vi "detElementContents.vi"(8 "error in (no error)":errorcluster, 10 "XMLString in":string, 11 "Element in":refnum<class "XMLParser.lvclass">) -> (0 "error out":errorcluster, 3 "Element out":refnum<class "XMLParser.lvclass">)   [LabVIEW 2014, in "XML.lvlib" / "XMLParser.lvclass"]
doc: "This method retrieves XML element contents of the XML input string."
uses:
  <userlib>/Common/XML/XMLParser/XMLParser.lvclass
  <userlib>/Common/XML/XMLParser/XMLParser.lvclass/XMLParser.ctl
  <vilib>/Utility/error.llb/Trim Whitespace.vi
  <userlib>/Common/XML/XMLAttributeParser/XMLAttributeParser.lvclass
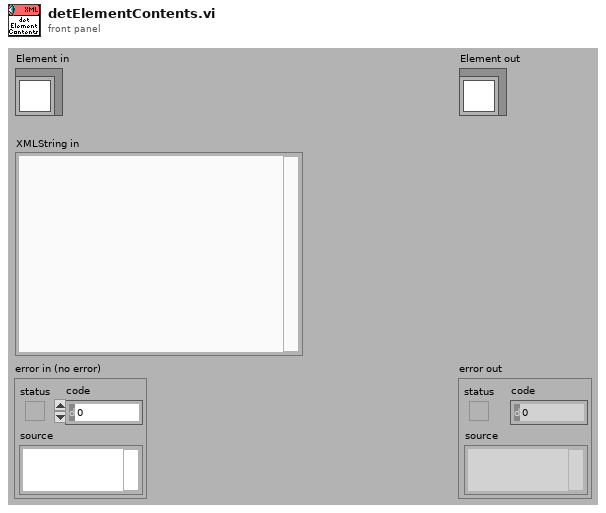
[diagram p1: front panel]
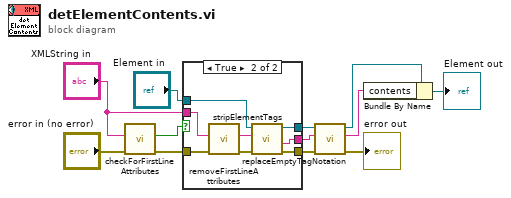
[diagram p0: block diagram]
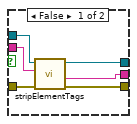
[diagram p2: hidden frame]
diagram:
  n1 = call <userlib>:"checkForFirstLineAttributes.vi"("error in (no error)"="error in (no error)", "XML In"="XMLString in") -> ("error out"=w10:errorcluster, "firstLineAttributeFound"=w8:bool)  [unwired: 7 in, 1 out]
  n2 = case shown="True" w8 {
    tunnel: [w17 w24] -> w7
    tunnel: "XMLString in" -> [w18 w26]
    tunnel: [w15 w21] -> w5
    tunnel: w10 -> [w16 w22]
    tunnel: "Element in" -> [w14 w20]
    tunnel: [w13 w19] -> w1
    frame False {
      n3 = call <userlib>:"stripElementTags.vi"("error in (no error)"=w16, "XMLContents In"=w18, "ReadElement in"=w14) -> ("error out"=w15:errorcluster, "Contents"=w17:string, "ReadElement out"=w13:refnum<class "XMLParser.lvclass">)  [unwired: 5 in, 1 out]
    }
    frame True {
      n4 = call <userlib>:"removeFirstLineAttributes.vi"("error in (no error)"=w22, "XMLString in"=w26) -> ("error out"=w23:errorcluster, "XMLString out"=w25:string)  [unwired: 8 in]
      n5 = call <userlib>:"stripElementTags.vi"("error in (no error)"=w23, "XMLContents In"=w25, "ReadElement in"=w20) -> ("error out"=w21:errorcluster, "Contents"=w24:string, "ReadElement out"=w19:refnum<class "XMLParser.lvclass">)  [unwired: 5 in, 1 out]
    }
  }
  n6 = call <userlib>:"replaceEmptyTagNotation.vi"("error in (no error)"=w5, "XML in"=w7, "ReadElement in"=w1) -> ("error out"=→"error out":errorcluster, "XML out"=w6:string, "ReadElement out"=w3:refnum<class "XMLParser.lvclass">)  [unwired: 6 in]
  n7 = Bundle By Name(cluster=w3, "contents"=w6) -> (→"Element out":refnum<class "XMLParser.lvclass">)
